vi "Encode Binary 1D Array Literal.vi"(1 "Array":bool[](array[boolean])) -> (0 "string":string)   [LabVIEW 2010, in "i3-json.lvlib"]
uses:
  i3-json.lvlib
  JSON Types/JSON Value String.ctl
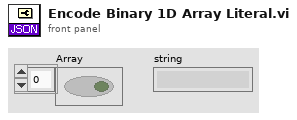
[diagram p1: front panel]
types:
  T1 = typedef "i3-json.lvlib/JSON Value String.ctl" = string
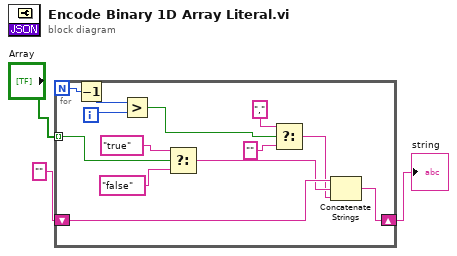
[diagram p0: block diagram]
diagram:
  n1 = for {
    N -> [w16]
    shift-right: [w4] -> w2
    shift-left: "" ("string") -> [w7]
    tunnel: "Array" -> [w13] mode=indexing
    i -> [w14]
    n2 = Decrement(x=w16) -> (x-1=w15:i32)
    n3 = Greater?(x=w15, y=w14) -> (0:w10:bool)
    n4 = Select(t=T1 "true" ("JSON Value String"), s=w13, f=T1 "false" ("JSON Value String")) -> (s? t:f=w6:T1)
    n5 = Select(t="," ("string"), s=w10, f="" ("string")) -> (s? t:f=w5:string)
    n6 = Concatenate Strings(w7, w6, w5) -> (w4:string)
  }
  "string" <- w2
